vi "Read TDMS.vi"(6 "Append Index":i32, 8 "error in (no error)":errorcluster, 11 "path":path) -> (0 "error out":errorcluster, 1 "Commands":string, 2 "Notes":string, 3 "Data (Dictionary)":T1[](array[typedef]))   [LabVIEW 2020, in "Data.TDMS.lvclass"]
uses:
  Data.TDMS.lvclass
  Data/Typedefs/Dictionary--cluster.ctl
  Data/Data.lvclass
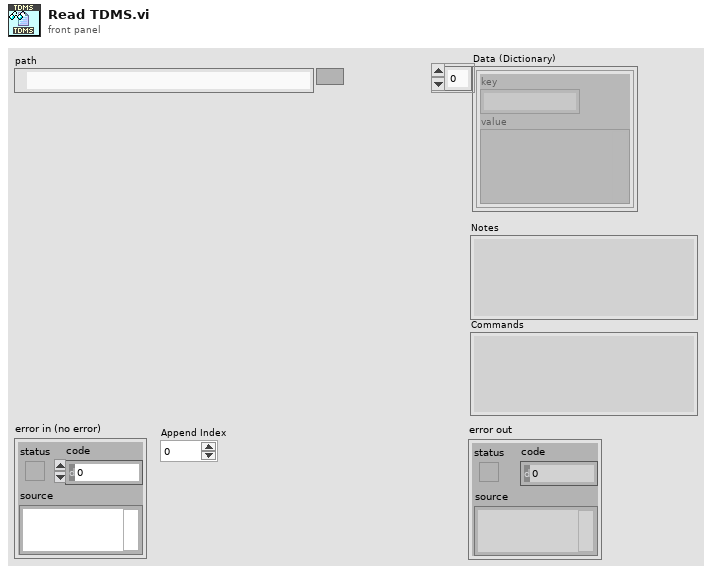
[diagram p1: front panel]
types:
  T1 = typedef "Data.lvclass/Dictionary--cluster.ctl" = cluster{"key":string, "value":variant}
  T2 = enum16{"open", "open or create", "create or replace", "create", "open (read-only)"}
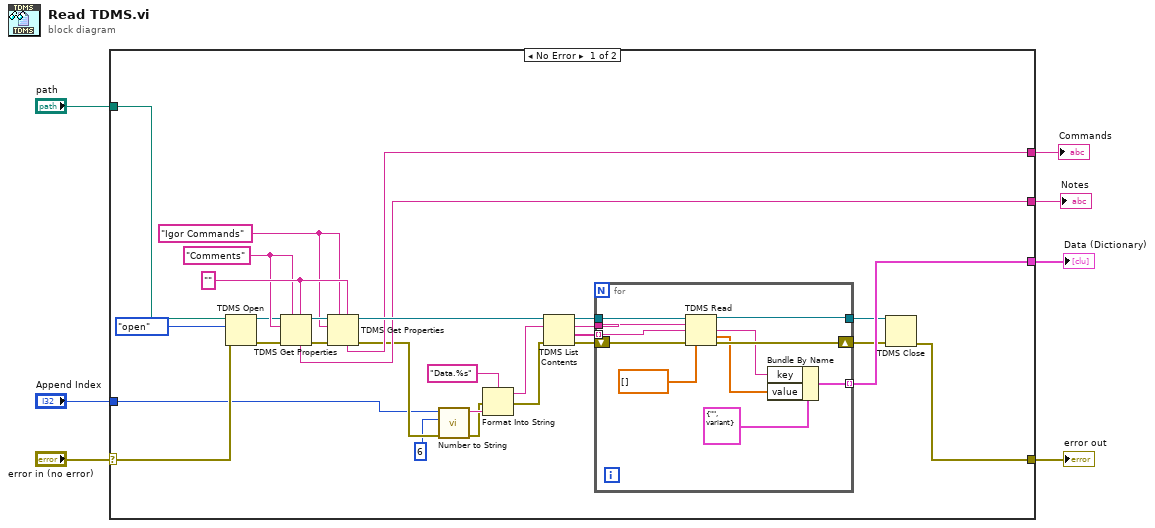
[diagram p0: block diagram]
diagram:
  n1 = case shown="No Error" "error in (no error)" {
    selector: "error in (no error)" -> [w14 w47]
    tunnel: [w9 w47] -> w6
    tunnel: "path" -> [w15 _]
    tunnel: [w26 _] -> w4
    tunnel: [w25 _] -> w3
    tunnel: [w24 _] -> w2
    tunnel: "Append Index" -> [w8 _]
    frame No Error {
      w36 = "" ("attrib name")
      w29 = "Igor Commands" ("attrib name")
      w30 = "Comments" ("attrib name")
      n2 = TDMS Open(8:w14, 10:T2."open" ("operation (0:open)"), 11:w15) -> (0:w12:errorcluster, 3:w13:refnum<k34>)  [unwired: 4 in]
      n3 = TDMS Get Properties(5:w36, 7:w30, 8:w12, 10:w30, 11:w13) -> (0:w33:errorcluster, 3:w34:refnum<k34>, 4:w24:string)  [unwired: 1 in, 3 out]
      n4 = TDMS Get Properties(5:w36, 7:w29, 8:w33, 10:w29, 11:w34) -> (0:w19:errorcluster, 3:w35:refnum<k34>, 4:w25:string)  [unwired: 1 in, 3 out]
      n5 = call <userlib>:"Number to String.vi"("error in (no error)"=w19, "desired minimum string length"=6, "Number"=w8) -> ("error out"=w18:errorcluster, "String"=w23:string)  [unwired: 7 in]
      n6 = Format Into String(format string="Data.%s", error in=w18, w23) -> (resulting string=w22:string, error out=w20:errorcluster)  [unwired: 1 in]
      n7 = TDMS List Contents(4:w20, 6:w22, 7:w35) -> (0:w31:errorcluster, 1:w27:string[], 2:w28:string, 3:w32:refnum<k34>)
      n8 = for {
        shift-right: [w43] -> w10
        shift-left: w31 -> [w46]
        tunnel: w27 -> [w38] mode=indexing
        tunnel: w28 -> [w42]
        tunnel: [w41] -> w26 mode=indexing
        tunnel: w32 -> [w44]
        tunnel: [w45] -> w11
        n9 = TDMS Read(0:w44, 5:w42, 7:w38, 11:w46, 12:dbl[] [] ("array type (2D Dbl)")) -> (4:w45:refnum<k34>, 10:w37:dbl[], 15:w43:errorcluster)  [unwired: 3 in, 3 out]
        n10 = Bundle By Name(cluster=T1 {"key"="", "value"=variant} ("key-value"), "key"=w38, "value"=w37) -> (w41:T1)
      }
      n11 = TDMS Close(8:w10, 11:w11) -> (0:w9:errorcluster)  [unwired: 1 out]
    }
    frame Error {
    }
  }
  "error out" <- w6
  "Data (Dictionary)" <- w4
  "Commands" <- w3
  "Notes" <- w2
